vi "DO_Write.vi"(0 "reference in":refnum<class "DO.lvclass">, 2 "Stop DO":bool, 3 "error in (no error)":errorcluster) -> (7 "reference out":refnum<class "DO.lvclass">, 10 "error out":errorcluster)   [LabVIEW 2017, in "DO.lvclass"]
uses:
  DO.lvclass
panel:
  # "This VI is called Asynchronously and will have one instance in memory\nfor each asynchronous call."
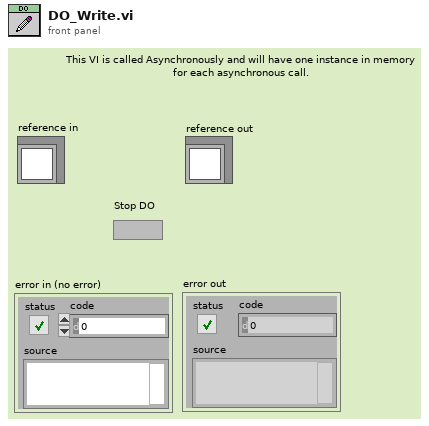
[diagram p1: front panel]
types:
  T1 = typedef "DO.lvclass/ObjectAttributes.ctl" = cluster{"DO Task":refnum<k21>, "DO Module Names (NI-Max Name)":string[], "Number of Channels Per DO Module":i32[], "DO Status":bool[], "Number of DO Modules":u32, "DO Status to Set":bool[], "DO On/Off Status":bool, "DO VI Reference":refnum<vi>, "Number of Total DO Channels":u32}
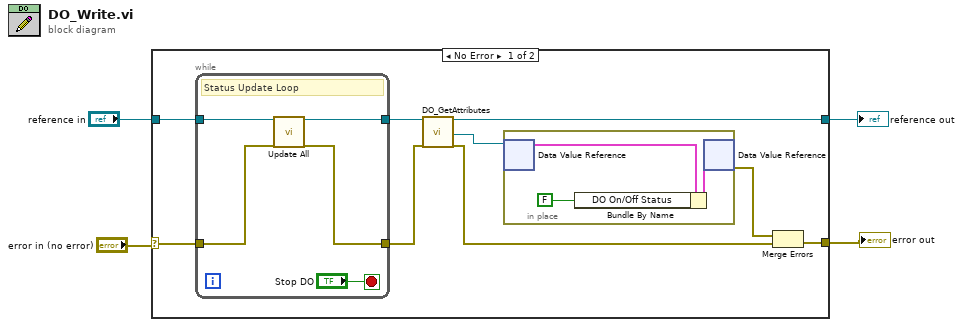
[diagram p0: block diagram]
diagram:
  n1 = case shown="No Error" "error in (no error)" {
    selector: "error in (no error)" -> [w13 w22]
    tunnel: [w5 w22] -> w3
    tunnel: "reference in" -> [w12 _]
    tunnel: [w10 _] -> w1
    frame No Error {
      n2 = while {
        tunnel: w13 -> [w16]
        tunnel: [w15] -> w7
        tunnel: w12 -> [w17]
        tunnel: [w14] -> w11
        stop <- "Stop DO" stop-if-true
        # "Status Update Loop"
        n3 = call-dynamic "Update All.vi"("reference in"=w17, "error in (no error)"=w16) -> ("reference out"=w14:refnum<class "DO.lvclass">, "error out"=w15:errorcluster)  [unwired: 16 in]
      }
      n4 = call "DO_GetAttributes.vi"("reference in"=w11, "error in (no error)"=w7) -> ("reference out"=w10:refnum<class "DO.lvclass">, "DataRef"=w8:refnum<data-value>, "error out"=w6:errorcluster)  [unwired: 14 in, 1 out]
      n5 = in-place {
        n6 = in-place-dvr #1(w8) -> (w21:T1)  [unwired: 1 out]
        n7 = Bundle By Name(cluster=w21, "DO On/Off Status"=FALSE) -> (w20:T1)
        n8 = in-place-dvr #1(w20) -> (w9:errorcluster)  [unwired: 1 out]
      }
      n9 = Merge Errors(w9, w6) -> (w5:errorcluster)
    }
    frame Error {
    }
  }
  "reference out" <- w1
  "error out" <- w3
